vi "Write Correct Data.vi"(10 "DataIn":string, 11 "DataName":string) -> ()   [LabVIEW 2019]
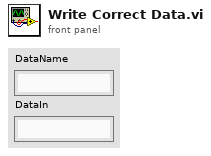
[diagram p1: front panel]
types:
  T1 = enum16{"Initial", "Write", "Read", "Save", "Load", "WrteAll"}
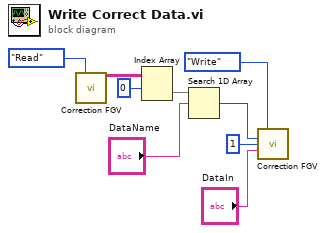
[diagram p0: block diagram]
diagram:
  n1 = call "Correction FGV.vi"("Action"=T1."Read") -> ("TableOut"=w9:string[][])  [unwired: 12 in, 2 out]
  n2 = Index Array(array=w9, index (row)=0) -> (element=w7:string[])  [unwired: 1 in]
  n3 = Search 1D Array(1D array=w7, element="DataName") -> (index of element=w5:i32)  [unwired: 1 in]
  n4 = call "Correction FGV.vi"("Action"=T1."Write", "X"=w5, "Y"=1, "DataIn"="DataIn") -> ()  [unwired: 9 in, 3 out]
